vi "Create-Traj-Benchmark.vi"() -> ()   [LabVIEW 2019]
uses:
  <vilib>/Rock Robotics/WPI/ThirdParty/JAS_Junk/TrajLib/Enum/TRAJECTORY_SPLINE_TYPE_ENUM.ctl
  <vilib>/Rock Robotics/WPI/ThirdParty/JAS_Junk/TrajLib/Translation2d_Create.vi
  <vilib>/Rock Robotics/WPI/ThirdParty/JAS_Junk/TrajLib/Rotation2d_CreateAngle.vi
  <vilib>/Rock Robotics/WPI/ThirdParty/JAS_Junk/TrajLib/Trajectory_Library.lvlib
panel:
  out "Quintic Time MS":dbl format="%18.3f"
  out "Cubic Time MS":dbl format="%18.3f"
  out "XY Graph":cluster{dbl[], dbl[]}[](graph)
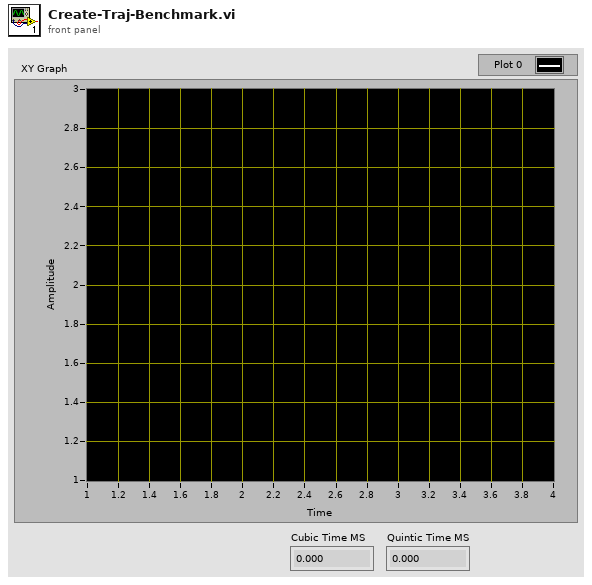
[diagram p1: front panel]
types:
  T1 = typedef "Trajectory_Library.lvlib/TRAJ_CONFIG.ctl" = cluster{"MaxVelocity":dbl, "Max Acceleration":dbl, "StartVelocity":dbl, "End Velocity":dbl, "Reversed":bool, "Constraints":variant[]}
  T2 = typedef "Trajectory_Library.lvlib/TRAJECTORY_SPLINE_TYPE_ENUM.ctl" = enum16{"Cubic", "Cubic With Weights", "Quintic", "Quintic With Weights"}
  T3 = typedef "Trajectory_Library.lvlib/WEIGHTED_WAYPOINT.ctl" = cluster{"TRANSLATION":T4, "ROTATION":T5, "SCALAR":dbl}
  T4 = typedef "Trajectory_Library.lvlib/TRANSLATION2D.ctl" = cluster{"X":dbl, "Y":dbl}
  T5 = typedef "Trajectory_Library.lvlib/ROTATION2D.ctl" = cluster{"VALUE":dbl, "COS":dbl, "SIN":dbl}
  T6 = typedef "Trajectory_Library.lvlib/TRAJECTORY.ctl" = cluster{"TotalTImeSecs":dbl, "States":T7[]}
  T7 = typedef "Trajectory_Library.lvlib/TRAJ_STATE.ctl" = cluster{"TimeSeconds":dbl, "Velocity":dbl, "Acceleration":dbl, "POSE":T8, "Curvature":dbl}
  T8 = typedef "Trajectory_Library.lvlib/POSE2D.ctl" = cluster{"TRANSLATION":T4, "ROTATION":T5}
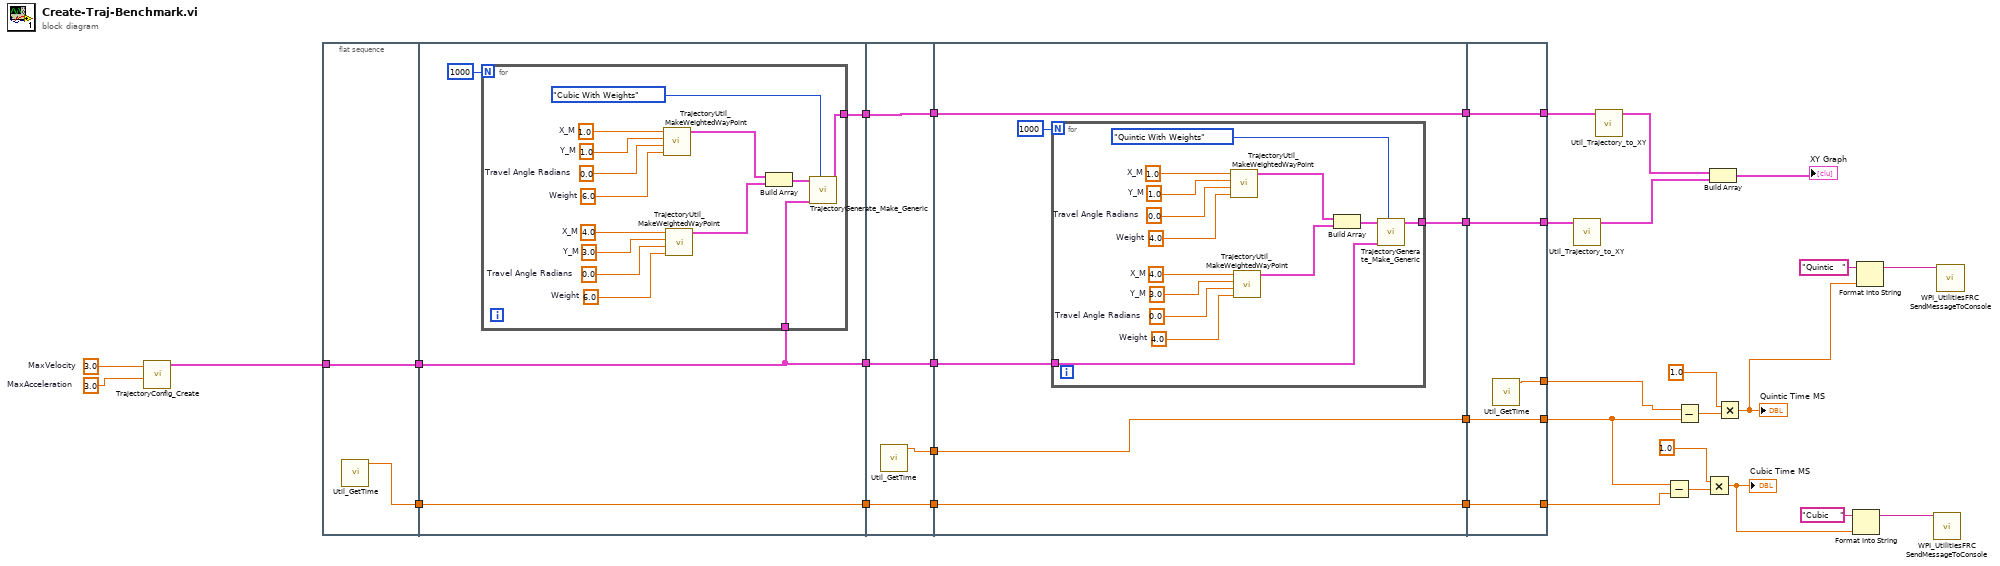
[diagram p0: block diagram]
diagram:
  w27 = 3.0  # MaxVelocity
  w28 = 3.0  # MaxAcceleration
  n1 = call <vilib>:"TrajectoryConfig_Create.vi"("MaxAcceleration"=w28, "MaxVelocity"=w27) -> ("TRAJECTORY_CONFIG"=w25:T1)  [unwired: 9 in]
  n2 = flat-sequence {
    tunnel: [w36] -> w32
    tunnel: [w35] -> w26
    tunnel: w25 -> [w35]
    tunnel: [w40] -> w33
    tunnel: w32 -> [w39]
    tunnel: [w39] -> w31
    tunnel: w26 -> [w38]
    tunnel: [w38] -> w21
    tunnel: w33 -> [w58]
    tunnel: w31 -> [w55]
    tunnel: [w58] -> w24
    tunnel: [w57] -> w23
    tunnel: [w56] -> w22
    tunnel: w21 -> [w56]
    tunnel: [w55] -> w12
    tunnel: w24 -> [w64]
    tunnel: w23 -> [w62]
    tunnel: w22 -> [w63]
    tunnel: [w64] -> w20
    tunnel: [w62] -> w16
    tunnel: [w61] -> w13
    tunnel: w12 -> [w61]
    tunnel: [w60] -> w10
    tunnel: [w83] -> w34
    tunnel: w20 -> [w83]
    tunnel: [w82] -> w17
    tunnel: [w81] -> w15
    tunnel: w16 -> [w81]
    tunnel: [w80] -> w14
    tunnel: w13 -> [w80]
    tunnel: [w79] -> w11
    tunnel: w10 -> [w79]
    frame #0 {
      n3 = call <vilib>:"Util_GetTime.vi"() -> ("FPGA_Time_Seconds"=w36:dbl)  [unwired: 10 in, 1 out]
    }
    frame #1 {
      n4 = for {
        N: 1000 -> [_]
        tunnel: [w43] -> w40
        tunnel: w38 -> [w41]
        w54 = 4.0  # X_M
        w53 = 3.0  # Y_M
        w52 = 0.0  # Travel Angle Radians
        w51 = 6.0  # Weight
        w50 = 1.0  # X_M
        w49 = 1.0  # Y_M
        w48 = 0.0  # Travel Angle Radians
        w47 = 6.0  # Weight
        n5 = call <vilib>:"TrajectoryUtil_MakeWeightedWayPoint.vi"("Weight"=w47, "Travel Angle Radians"=w48, "Y_M"=w49, "X_M"=w50) -> ("WEIGHTED_WAYPOINT"=w45:T3)  [unwired: 7 in]
        n6 = call <vilib>:"TrajectoryUtil_MakeWeightedWayPoint.vi"("Weight"=w51, "Travel Angle Radians"=w52, "Y_M"=w53, "X_M"=w54) -> ("WEIGHTED_WAYPOINT"=w44:T3)  [unwired: 7 in]
        n7 = Build Array(w45, w44) -> (w46:T3[])
        n8 = call <vilib>:"TrajectoryGenerate_Make_Generic.vi"("Spline Type"=TRAJECTORY_SPLINE_TYPE_ENUM."Cubic With Weights", "traj_config"=w41, "WeightedWayPoints"=w46) -> ("TRAJECTORY"=w43:T6)  [unwired: 7 in, 1 out]
      }
    }
    frame #2 {
      n9 = call <vilib>:"Util_GetTime.vi"() -> ("FPGA_Time_Seconds"=w57:dbl)  [unwired: 10 in, 1 out]
    }
    frame #3 {
      n10 = for {
        N: 1000 -> [_]
        tunnel: w63 -> [w66]
        tunnel: [w65] -> w60
        w78 = 4.0  # X_M
        w77 = 3.0  # Y_M
        w76 = 0.0  # Travel Angle Radians
        w75 = 4.0  # Weight
        w74 = 1.0  # X_M
        w73 = 1.0  # Y_M
        w72 = 0.0  # Travel Angle Radians
        w71 = 4.0  # Weight
        n11 = call <vilib>:"TrajectoryUtil_MakeWeightedWayPoint.vi"("Weight"=w71, "Travel Angle Radians"=w72, "Y_M"=w73, "X_M"=w74) -> ("WEIGHTED_WAYPOINT"=w69:T3)  [unwired: 7 in]
        n12 = call <vilib>:"TrajectoryUtil_MakeWeightedWayPoint.vi"("Weight"=w75, "Travel Angle Radians"=w76, "Y_M"=w77, "X_M"=w78) -> ("WEIGHTED_WAYPOINT"=w68:T3)  [unwired: 7 in]
        n13 = Build Array(w69, w68) -> (w70:T3[])
        n14 = call <vilib>:"TrajectoryGenerate_Make_Generic.vi"("Spline Type"=TRAJECTORY_SPLINE_TYPE_ENUM."Quintic With Weights", "traj_config"=w66, "WeightedWayPoints"=w70) -> ("TRAJECTORY"=w65:T6)  [unwired: 7 in, 1 out]
      }
    }
    frame #4 {
      n15 = call <vilib>:"Util_GetTime.vi"() -> ("FPGA_Time_Seconds"=w82:dbl)  [unwired: 10 in, 1 out]
    }
  }
  n16 = call <vilib>:"Util_Trajectory_to_XY.vi"("TRAJECTORY"=w11) -> ("outArrayXY"=w8:cluster{dbl[], dbl[]})  [unwired: 10 in]
  n17 = call <vilib>:"Util_Trajectory_to_XY.vi"("TRAJECTORY"=w34) -> ("outArrayXY"=w9:cluster{dbl[], dbl[]})  [unwired: 10 in]
  n18 = Subtract(x=w15, y=w14) -> (x-y=w30:dbl)
  n19 = Subtract(x=w17, y=w15) -> (x-y=w19:dbl)
  n20 = Multiply(x=1.0, y=w30) -> (x*y=w1:dbl)
  "Cubic Time MS" <- w1
  n21 = Build Array(w9, w8) -> (→"XY Graph":cluster{dbl[], dbl[]}[])
  n22 = Multiply(x=1.0, y=w19) -> (x*y=w5:dbl)
  "Quintic Time MS" <- w5
  n23 = Format Into String(initial string="Cubic    ", w1) -> (resulting string=w2:string)  [unwired: 2 in, 1 out]
  n24 = Format Into String(initial string="Quintic   ", w5) -> (resulting string=w4:string)  [unwired: 2 in, 1 out]
  n25 = call <vilib>:"WPI_UtilitiesFRC SendMessageToConsole.vi"("Message"=w2) -> ()  [unwired: 14 in, 1 out]
  n26 = call <vilib>:"WPI_UtilitiesFRC SendMessageToConsole.vi"("Message"=w4) -> ()  [unwired: 14 in, 1 out]
